vi "Connect.vi"(8 "error in":errorcluster, 11 "3300 in":refnum<class "3300.lvclass">) -> (0 "error out":errorcluster, 3 "3300 out":refnum<class "3300.lvclass">)   [LabVIEW 2019, in "3300.lvlib" / "3300.lvclass"]
uses:
  Library/3300.lvclass
  C:/Users/Public/Documents/Development/builds/Instruments/Instruments.lvlibp/Library/Instruments.lvclass
  Library/3300.lvclass/3300.ctl
  builds/Instruments/Instruments.lvlibp/Accessors/Read Resource.vi
  <instrlib>/Agilent N330X Series/Agilent N330X Series.lvlib
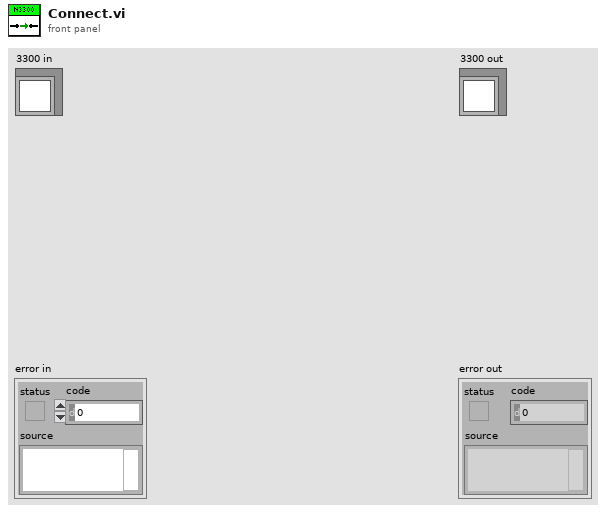
[diagram p1: front panel]
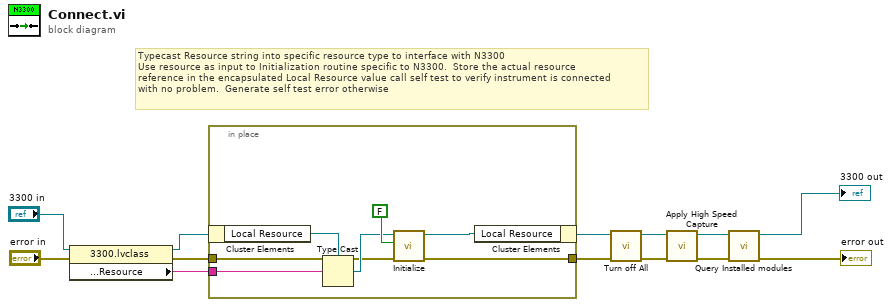
[diagram p0: block diagram]
diagram:
  # "Typecast Resource string into specific resource type to interface with N3300\nUse resource as input to Initialization routine specific to N3300.  Store the actual resource\nreference in the encapsulated Local Resource value call self test to verify instrument is connected\nwith no problem.  Generate self test error otherwise"
  n1 = property class="3300.lvclass"(reference="3300 in", error in="error in") -> (reference out=w10:refnum<class "3300.lvclass">, error out=w11:errorcluster, "Accessors:Configuration:Resource"=w9:string)
  n2 = in-place {
    in-place-border: w11 -> [w16]
    in-place-border: w9 -> [w19]
    in-place-border: [w14] -> w3
    n3 = in-place-cluster #1(w10) -> ("Local Resource"=w20:refnum<visa-resource-name>)
    n4 = Type Cast(type=w20, x=w19) -> (*(type *) &x=w17:refnum<visa-resource-name>)
    n5 = call <instrlib>:"Initialize.vi"("error in (no error)"=w16, "ID Query (True)"=FALSE, "VISA resource name"=w17) -> ("error out"=w14:errorcluster, "VISA resource name out"=w15:refnum<visa-resource-name>)  [unwired: 7 in]
    n6 = in-place-cluster #1("Local Resource"=w15) -> (w4:refnum<class "3300.lvclass">)
  }
  n7 = call-dynamic "Turn off All.vi"("error in"=w3, "3300 in"=w4) -> ("error out"=w1:errorcluster, "3300 out"=w2:refnum<class "3300.lvclass">)  [unwired: 8 in]
  n8 = call "Apply High Speed Capture.vi"("error in"=w1, "3300 in"=w2) -> ("error out"=w8:errorcluster, "3300 out"=w7:refnum<class "3300.lvclass">)  [unwired: 8 in]
  n9 = call "Query Installed modules.vi"("error in"=w8, "3300 in"=w7) -> ("error out"=→"error out":errorcluster, "3300 out"=→"3300 out":refnum<class "3300.lvclass">)  [unwired: 8 in]
